vi "Setup Multi Acq.vi"(6 "# of Scans":u32, 7 "Time Between Acq (ms)":u32, 8 "Cosmic Ray Removal?":bool, 9 "Averaging?":bool, 10 "Dark Subtract?":bool, 11 "Synapse CCD.lvclass In":refnum<class "Synapse CCD.lvclass">) -> (3 "Synapse CCD.lvclass Out":refnum<class "Synapse CCD.lvclass">)   [LabVIEW 2017, in "Synapse CCD.lvclass"]
doc: "Loads Multi-Acq parameters into member data and creates Boolean Control Array for member data."
uses:
  Synapse CCD.lvclass
  Synapse CCD.lvclass/Synapse CCD.ctl
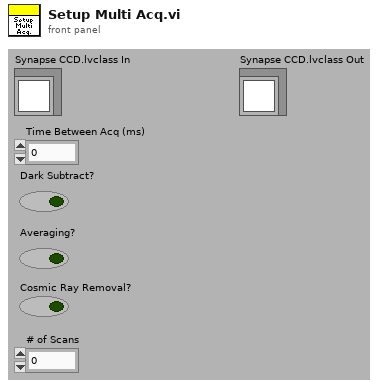
[diagram p1: front panel]
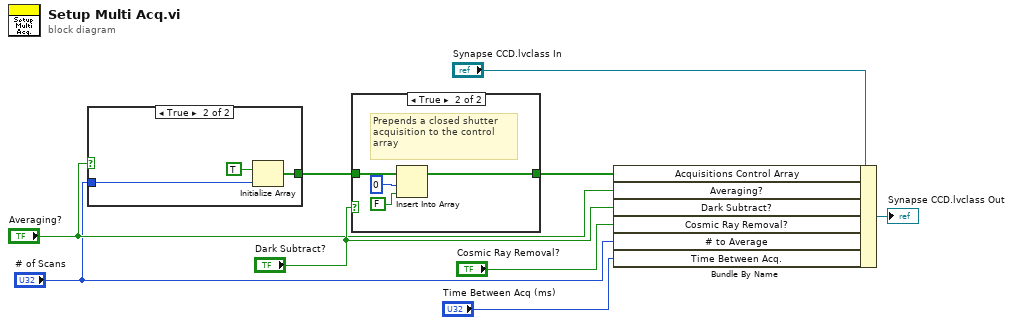
[diagram p0: block diagram]
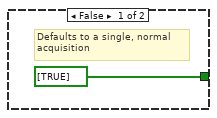
[diagram p3: hidden frame]
diagram:
  n1 = case shown="True" "Averaging?" {
    tunnel: [bool[] [TRUE] w12] -> w9
    tunnel: "# of Scans" -> [_ w11]
    frame False {
      # "Defaults to a single, normal\nacquisition"
    }
    frame True {
      n2 = Initialize Array(TRUE, w11) -> (w12:bool[])
    }
  }
  n3 = case shown="True" "Dark Subtract?" {
    tunnel: w9 -> [w14 w18]
    tunnel: [w14 w15] -> w6
    frame False {
    }
    frame True {
      # "Prepends a closed shutter\nacquisition to the control\narray"
      n4 = Insert Into Array(array=w18, index=0, new element=FALSE) -> (w15:bool[])
    }
  }
  n5 = Bundle By Name(cluster="Synapse CCD.lvclass In", "Acquisitions Control Array"=w6, "Averaging?"="Averaging?", "Dark Subtract?"="Dark Subtract?", "Cosmic Ray Removal?"="Cosmic Ray Removal?", "# to Average"="# of Scans", "Time Between Acq."="Time Between Acq (ms)") -> (→"Synapse CCD.lvclass Out":refnum<class "Synapse CCD.lvclass">)
